vi "setSerializedData.vi"(0 "reference":refnum<class "AbstractEdge.lvclass">, 1 "startNode":refnum<class "AbstractNode.lvclass">, 2 "endNode":refnum<class "AbstractNode.lvclass">, 3 "xmlOut":string, 5 "error in (no error)":errorcluster) -> (14 "reference out":refnum<class "AbstractEdge.lvclass">, 19 "error out":errorcluster)   [LabVIEW 2012, in "AbstractEdge.lvclass"]
doc: "Sets data"
uses:
  <resource>/Framework/Providers/Open_GDS/UML/AbstractEdge_class/AbstractEdge.lvclass
  <resource>/Framework/Providers/Open_GDS/UML/AbstractNode_class/AbstractNode.lvclass
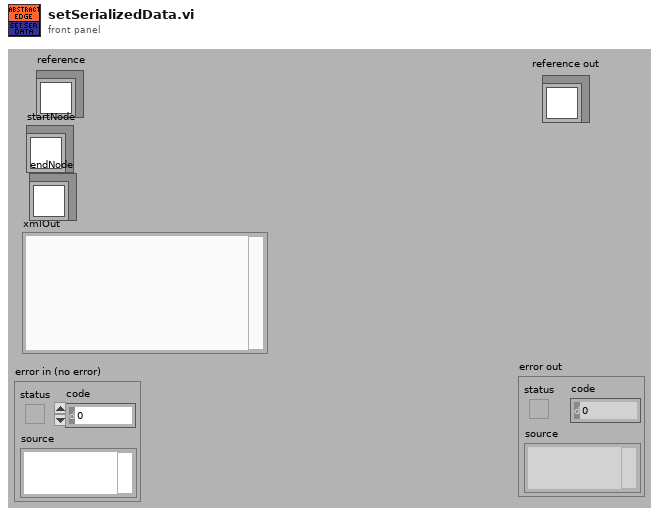
[diagram p1: front panel]
types:
  T1 = typedef "AbstractEdge.lvclass/ObjectAttributes.ctl" = cluster{"start":refnum<class "AbstractNode.lvclass">, "end":refnum<class "AbstractNode.lvclass">}
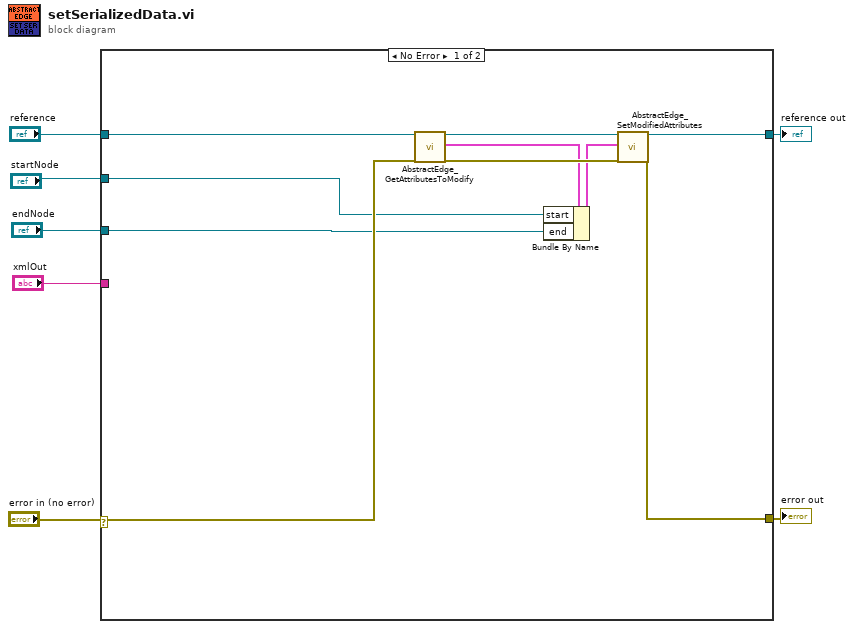
[diagram p0: block diagram]
diagram:
  n1 = case shown="No Error" "error in (no error)" {
    selector: "error in (no error)" -> [w14 w17]
    tunnel: "reference" -> [w16 w18]
    tunnel: [w15 w17] -> w6
    tunnel: [w16 w18] -> w5
    tunnel: "startNode" -> [w13 _]
    tunnel: "endNode" -> [w12 _]
    tunnel: "xmlOut" -> [_ _]
    frame No Error {
      n2 = call <resource>:"AbstractEdge_GetAttributesToModify.vi"("reference in"=w16, "error in (no error)"=w14) -> ("reference out"=w10:refnum<class "AbstractEdge.lvclass">, "Attributes"=w9:T1, "error out"=w11:errorcluster)  [unwired: 1 in, 14 out]
      n3 = Bundle By Name(cluster=w9, "start"=w13, "end"=w12) -> (w8:T1)
      n4 = call <resource>:"AbstractEdge_SetModifiedAttributes.vi"("reference in"=w10, "Attributes"=w8, "error in (no error)"=w11) -> ("error out"=w15:errorcluster)  [unwired: 3 in, 13 out]
    }
    frame Error {
    }
  }
  "reference out" <- w5
  "error out" <- w6
